vi "Initialize_SVs.vi"(8 "error in (no error)":errorcluster, 11 "error in":errorcluster) -> (0 "error out":errorcluster, 3 "error IO":errorcluster)   [LabVIEW 2017]
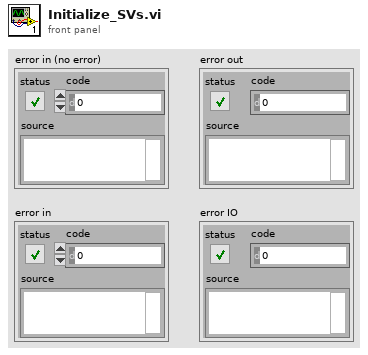
[diagram p1: front panel]
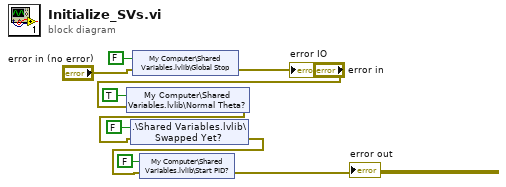
[diagram p0: block diagram]
diagram:
  n1 = shared-variable "My Computer\\Shared Variables.lvlib\\Normal Theta?"(TRUE ("Add 360?"), error in="error in") -> (error out=w4:errorcluster)
  n2 = shared-variable ".\\Shared Variables.lvlib\\Swapped Yet?"(FALSE ("Swapped Yet?"), error in=w4) -> (error out=w10:errorcluster)
  n3 = shared-variable "My Computer\\Shared Variables.lvlib\\Global Stop"(FALSE ("Global Stop"), error in="error in (no error)") -> (error out=→"error IO":errorcluster)
  n4 = shared-variable "My Computer\\Shared Variables.lvlib\\Start PID?"(FALSE ("Start PID?"), error in=w10) -> (error out=→"error out":errorcluster)
